vi "ROS_Master_lookupNodeReply.vi"(2 "node":string, 3 "ROS_Master in":T1) -> (0 "XML":string)   [LabVIEW 2014]
doc: "Returns XML from registering a node with the master"
uses:
  <userlib>/ROS for LabVIEW Software/ROS/Code/ROS_Master/ROS_Master.ctl
  <userlib>/ROS for LabVIEW Software/ROS/Code/ROS_Master/ROS_Topic.ctl
  <userlib>/ROS for LabVIEW Software/ROS/Code/ROS_Master/ROS_Node.ctl
  <userlib>/ROS for LabVIEW Software/ROS/Code/ROS_Master/ROS_Service.ctl
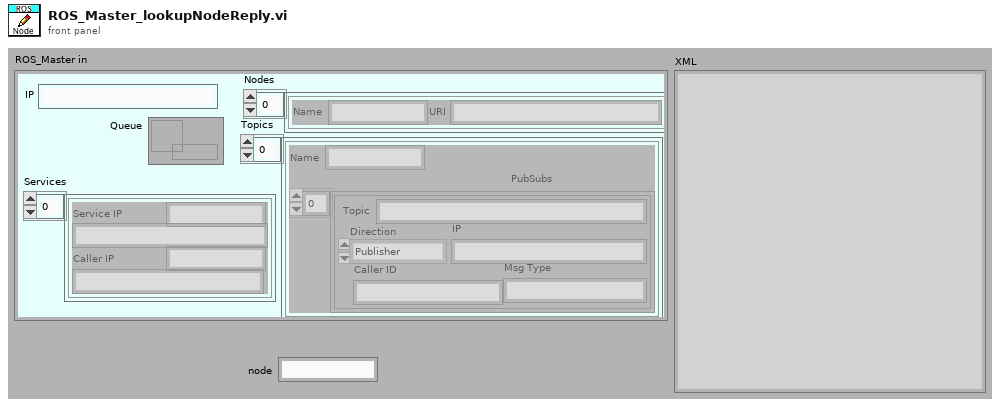
[diagram p1: front panel]
types:
  T1 = typedef "ROS_Master.ctl" = cluster{"IP":string, "Topics":cluster{"Name":string, "PubSubs":T2[]}[], "Nodes":T3[], "Services":T4[], "Queue":refnum<queue>}
  T2 = typedef "ROS_Topic.ctl" = cluster{"Caller ID":string, "IP":string, "Msg Type":string, "Direction":enum16{"Publisher", "Subscriber"}, "Topic":string}
  T3 = typedef "ROS_Node.ctl" = cluster{"Name":string, "URI":string}
  T4 = typedef "ROS_Service.ctl" = cluster{"Service":string, "Service IP":string, "Caller IP":string, "Caller ID":string}
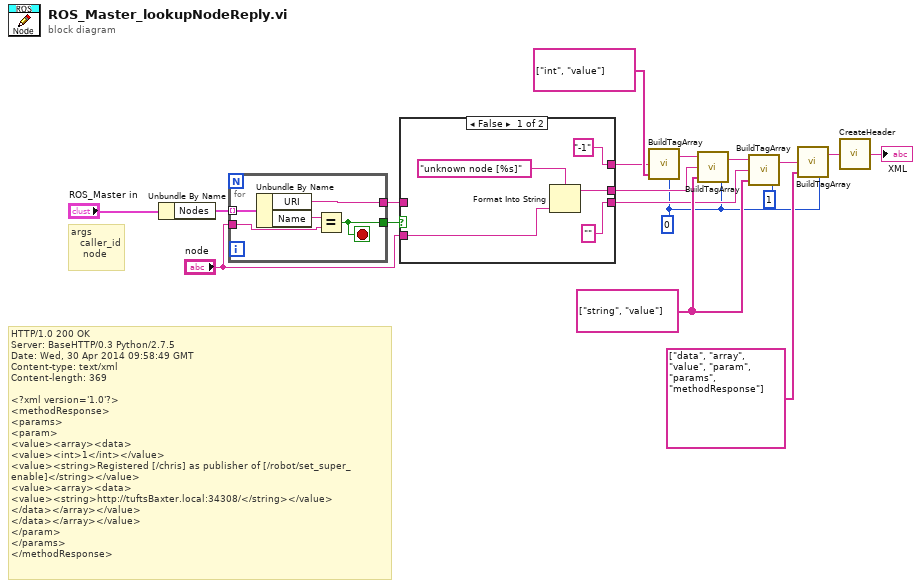
[diagram p0: block diagram]
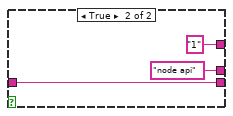
[diagram p2: hidden frame]
diagram:
  w2 = i8 0 ("Indent")
  w9 = string[] ["string", "value"] ("tags")
  # "args\n   caller_id\n    node"
  # "HTTP/1.0 200 OK\nServer: BaseHTTP/0.3 Python/2.7.5\nDate: Wed, 30 Apr 2014 09:58:49 GMT\nContent-type: text/xml\nContent-length: 369\n\n<?xml version='1.0'?>\n<methodResponse>\n<params>\n<param>\n<value><array><data>\n<value><int>1</int></value>\n<value><string>Registered [/chris] as publisher of [/robot/set_super_enable]</string></value>\n<value><array><data>\n<value><string>http://tuftsBaxter.local:34308/</string></value>\n</data></array></value>\n</data></array></value>\n</param>\n</params>\n</methodResponse>"
  n1 = Unbundle By Name("ROS_Master in") -> ("Nodes"=w13:T3[])
  n2 = for {
    tunnel: w13 -> [w23] mode=indexing
    tunnel: "node" -> [w21]
    tunnel: [w20] -> w12
    tunnel: [w19] -> w11
    stop <- w20 stop-if-true
    n3 = Unbundle By Name(w23) -> ("URI"=w19:string, "Name"=w22:string)
    n4 = Equal?(x=w22, y=w21) -> (x = y?=w20:bool)
  }
  n5 = case shown="False" w12 {
    tunnel: w11 -> [_ w30]
    tunnel: "node" -> [w26 _]
    tunnel: ["-1" ("value") "1" ("value")] -> w7
    tunnel: ["" ("URI") w30] -> w6
    tunnel: [w25 "node api" ("value")] -> w5
    frame False {
      n6 = Format Into String(format string="unknown node [%s]", w26) -> (resulting string=w25:string)  [unwired: 2 in, 1 out]
    }
    frame True {
    }
  }
  n7 = call <userlib>:"BuildTagArray.vi"("Indent"=w2, "tags"=string[] ["int", "value"], "value"=w7) -> ("string out"=w17:string)  [unwired: 1 in]
  n8 = call <userlib>:"BuildTagArray.vi"("Indent"=w2, "tags"=w9, "value"=w5, "string in"=w17) -> ("string out"=w8:string)
  n9 = call <userlib>:"BuildTagArray.vi"("Indent"=i8 1, "tags"=w9, "value"=w6, "string in"=w8) -> ("string out"=w4:string)
  n10 = call <userlib>:"BuildTagArray.vi"("Indent"=w2, "tags"=string[] ["data", "array", "value", "param", "params", "methodResponse"], "value"=w4) -> ("string out"=w15:string)  [unwired: 1 in]
  n11 = call <userlib>:"CreateHeader.vi"("Content"=w15) -> ("XML"=→"XML":string)
